vi "FTW-Publisher-Destroy.vi"(0 "FTW Publisher":refnum<data-value>, 11 "error in":errorcluster) -> (15 "error out":errorcluster)   [LabVIEW 2014]
uses:
  core/FTW-Publisher-Core-Type.ctl
  error/FTW-ERR-ThrowGenericError.vi
  error/FTW-ERR-ThrowError.vi
  error/FTW-ERR-CallChain.vi
  string/FTW-STR-ReplaceWhitespace.vi
panel:
  # "Inputs"
  # "Outputs"
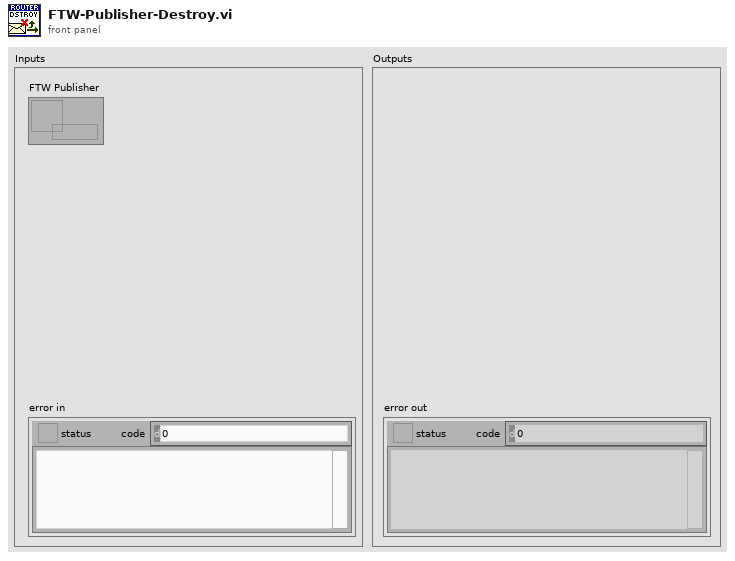
[diagram p1: front panel]
types:
  T1 = typedef "FTW-Publisher-Core-Type.ctl" = cluster{"Socket":i64}
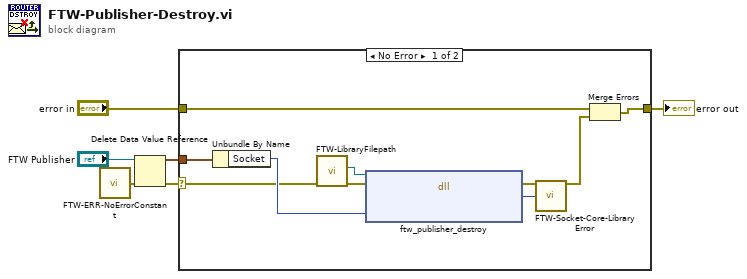
[diagram p0: block diagram]
diagram:
  n1 = call "FTW-ERR-NoErrorConstant.vi"() -> ("no error"=w1:errorcluster)
  n2 = Delete Data Value Reference(data value reference="FTW Publisher", error in=w1) -> (data value=w3:T1, error out=w2:errorcluster)
  n3 = case shown="No Error" w2 {
    selector: w2 -> [w7 _]
    tunnel: [w16 w17] -> w6
    tunnel: "error in" -> [w14 w17]
    tunnel: w3 -> [w12 _]
    frame No Error {
      n4 = Unbundle By Name(w12) -> ("Socket"=w13:i64)
      n5 = call "FTW-LibraryFilepath.vi"("error in"=w7) -> ("error out"=w8:errorcluster, "Library Filepath"=w11:path)  [unwired: 8 in, 1 out]
      n6 = dll-call lib="C:/Users/Jack/repo/ftw-master/Actor/src/Endpoint/Core/FTWLib-nanomsg32.dll" fn="ftw_publisher_destroy"(path in=w11, error in=w8, "Socket"=w13) -> (error out=w10:errorcluster, "Return Value"=w9:i64)  [unwired: 2 in, 1 out]
      n7 = call "FTW-Socket-Core-LibraryError.vi"("error in"=w10, "Return Value"=w9) -> ("error out"=w15:errorcluster)  [unwired: 13 in]
      n8 = Merge Errors(w14, w15) -> (w16:errorcluster)
    }
    frame Error {
    }
  }
  "error out" <- w6
